vi "sav_dat2db.vi"(4 "Slide Ref":refnum<vi>, 6 "error in":errorcluster, 8 "Array":cluster{"x0":dbl, "dx":dbl, "y":sgl[][]}[](array[cluster]), 9 "date/time":timestamp) -> (1 "error out":errorcluster)   [LabVIEW 2010]
uses:
  <vilib>/addons/database/Auxilliary.llb/DB Tools Column Info.ctl
  <vilib>/addons/database/Auxilliary.llb/DB Tools DataTypes.ctl
  70user.lib/TheSigTab.vi
  <vilib>/addons/database/NI_Database_API.lvlib
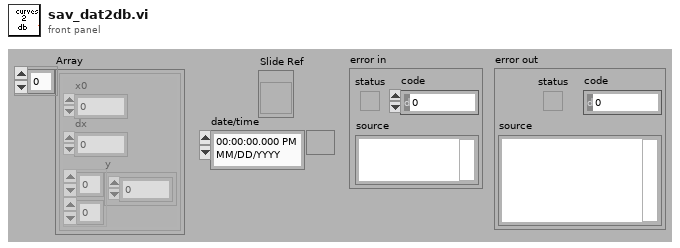
[diagram p1: front panel]
types:
  T1 = cluster{"type":string, "units":string, "n":i32}[]
  T2 = enum16{"Напряжение/Ток", "ЧР", "Температура", "Давление"}
  T3 = typedef "NI_Database_API.lvlib/DB Tools Column Info.ctl" = cluster{"column name":string, "data type":T4, "size":i32, "allow null?":bool}
  T4 = typedef "NI_Database_API.lvlib/DB Tools DataTypes.ctl" = enum16{"String", "Long (I32)", "Single (SGL)", "Double (DBL)", "Date/Time", "Binary"}
  T5 = typedef "NI_Database_API.lvlib/Conn ObjectReference.ctl" = refnum<k1>
  T6 = cluster{"Сигнал":string, "Тип":enum16{"Напряжение/Ток", "ЧР", "Температура", "Давление"}, "Object":string}[]
  T7 = cluster{"Сигнал":string, "Тип":enum16{"Напряжение/Ток", "ЧР", "Температура", "Давление"}, "Object":string}
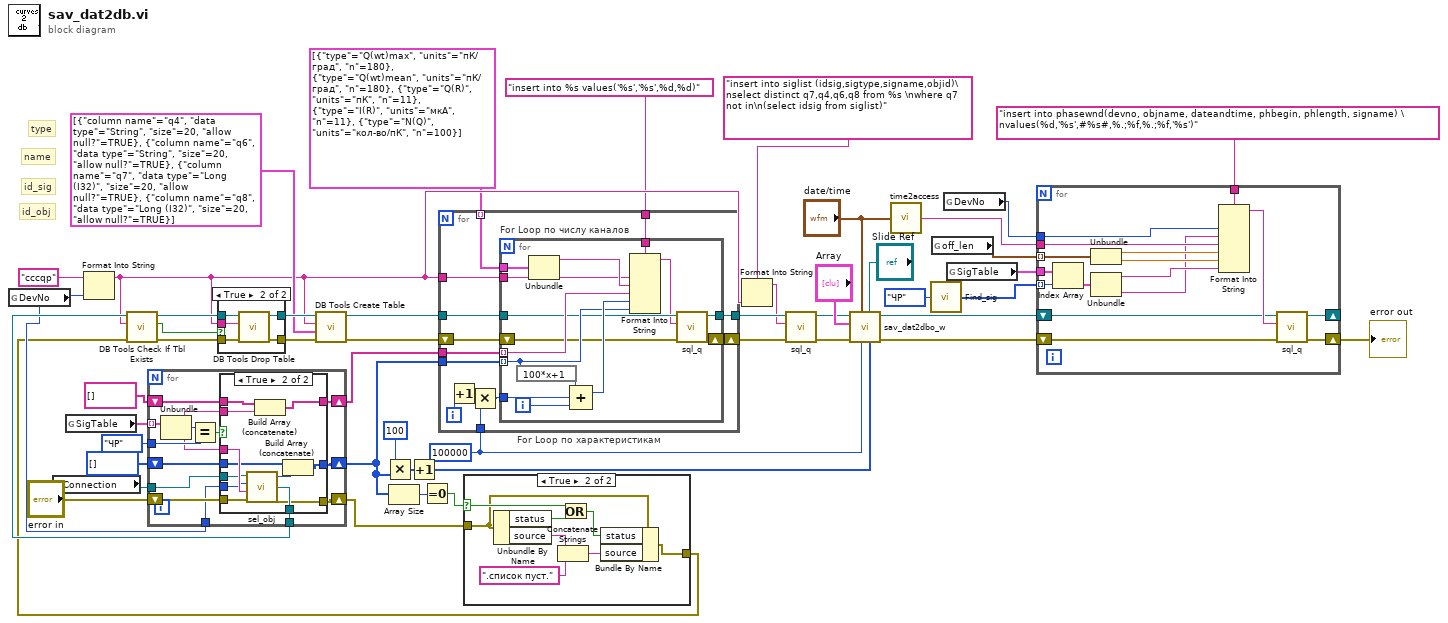
[diagram p0: block diagram]
diagram:
  w23 = 100000
  # "id_obj"
  # "id_sig"
  # "type"
  # "name"
  n1 = global read "TheSigTab.vi" "DevNo"() -> (w10:u32)
  n2 = global read "TheSigTab.vi" "Connection"() -> (w28:T5)
  n3 = global read "TheSigTab.vi" "SigTable"() -> (w48:T6)
  n4 = Format Into String(initial string="cccqp", w10) -> (resulting string=w31:string)  [unwired: 2 in, 1 out]
  n5 = for {
    tunnel: w48 -> [w59] mode=indexing
    shift-right: [w63] -> w46
    shift-left: string[] [] ("columns") -> [w62]
    tunnel: T2."ЧР" ("Тип") -> [w60]
    shift-right: [w56] -> w17
    shift-left: i32[] [] -> [w55]
    tunnel: w28 -> [w54]
    tunnel: [w53] -> w36
    shift-right: [w52] -> w1
    shift-left: "error in" -> [w51]
    tunnel: w10 -> [w50]
    n6 = Unbundle(w59) -> ("Сигнал"=w58:string, "Тип"=w64:T2, "Object"=w57:string)
    n7 = Equal?(x=w64, y=w60) -> (x = y?=w61:bool)
    n8 = case shown="True" w61 {
      tunnel: [w68 w80] -> w63
      tunnel: w62 -> [w68 w79]
      tunnel: w58 -> [_ w78]
      tunnel: w57 -> [_ w77]
      tunnel: [w67 w75] -> w56
      tunnel: w55 -> [w67 w74]
      tunnel: w54 -> [w66 w73]
      tunnel: [w66 w72] -> w53
      tunnel: [w65 w71] -> w52
      tunnel: w51 -> [w65 w70]
      tunnel: w50 -> [_ w69]
      frame False {
      }
      frame True {
        n9 = call "sel_obj.vi"("error in"=w70, "Object"=w77, "DevNo"=w69, "conn ref in"=w73) -> ("error out"=w71:errorcluster, "conn ref out"=w72:T5, "Obj Id"=w76:i32)
        n10 = Build Array (concatenate)(w79, w78) -> (w80:string[])
        n11 = Build Array (concatenate)(w74, w76) -> (w75:i32[])
      }
    }
  }
  n12 = Multiply(x=100, y=w17) -> (x*y=w44:i32[])
  n13 = Array Size(array=w17) -> (size(s)=w16:i32)
  n14 = Increment(x=w44) -> (x+1=w22:i32[])
  n15 = Equal To 0?(x=w16) -> (x = 0?=w2:bool)
  n16 = case shown="True" w2 {
    selector: w2 -> [_ w88]
    tunnel: [w81 w89] -> w3
    tunnel: w1 -> [w81 w86]
    frame False {
    }
    frame True {
      n17 = Unbundle By Name(w86) -> ("status"=w87:bool, "source"=w83:string)
      n18 = Concatenate Strings(w83, ".список пуст." ("source")) -> (w84:string)
      n19 = Or(x=w88, y=w87) -> (x .or. y?=w85:bool)
      n20 = Bundle By Name(cluster=w86, "status"=w85, "source"=w84) -> (w89:errorcluster)
    }
  }
  n21 = call <vilib>:"DB Tools Check If Tbl Exists.vi"("error in (no error)"=w3, "table name"=w31, "connection reference"=w36) -> ("error out"=w33:errorcluster, "exists?"=w34:bool, "connection reference out"=w35:T5)  [unwired: 2 in]
  n22 = case shown="True" w34 {
    tunnel: [w91 w96] -> w43
    tunnel: w31 -> [_ w95]
    tunnel: w35 -> [w91 w94]
    tunnel: w33 -> [w90 w93]
    tunnel: [w90 w92] -> w42
    frame False {
    }
    frame True {
      n23 = call <vilib>:"DB Tools Drop Table.vi"("error in (no error)"=w93, "table"=w95, "connection reference"=w94) -> ("error out"=w92:errorcluster, "connection reference out"=w96:T5)  [unwired: 5 in]
    }
  }
  n24 = call <vilib>:"DB Tools Create Table.vi"("error in (no error)"=w42, "column information"=T3[] [{"column name"="q4", "data type"=enum."String", "size"=20, "allow null?"=TRUE}, {"column name"="q6", "data type"=enum."String", "size"=20, "allow null?"=TRUE}, {"column name"="q7", "data type"=enum."Long (I32)", "size"=20, "allow null?"=TRUE}, {"column name"="q8", "data type"=enum."Long (I32)", "size"=20, "allow null?"=TRUE}], "table"=w31, "connection reference"=w43) -> ("error out"=w41:errorcluster, "connection reference out"=w40:T5)  [unwired: 4 in]
  n25 = for "For Loop по характеристикам" {
    shift-right: [w109] -> w20
    shift-left: w41 -> [w108]
    tunnel: w46 -> [w107]
    tunnel: w23 -> [w105]
    tunnel: w40 -> [w103]
    tunnel: w31 -> [w102]
    tunnel: [w101] -> w21
    tunnel: w17 -> [w100]
    tunnel: T1 [{"type"="Q(wt)max", "units"="пК/град", "n"=180}, {"type"="Q(wt)mean", "units"="пК/град", "n"=180}, {"type"="Q(R)", "units"="пК", "n"=11}, {"type"="I(R)", "units"="мкА", "n"=11}, {"type"="N(Q)", "units"="кол-во/пК", "n"=100}] -> [w98] mode=indexing
    tunnel: "insert into %s values('%s','%s',%d,%d)" -> [w97]
    i -> [w106]
    n26 = Increment(x=w106) -> (x+1=w104:i32)
    n27 = Multiply(x=w104, y=w105) -> (x*y=w99:i32)
    n28 = for "For Loop по числу каналов" {
      shift-right: [w113] -> w109
      shift-left: w108 -> [w112]
      tunnel: w107 -> [w120] mode=indexing
      tunnel: w103 -> [w115]
      tunnel: w102 -> [w116]
      tunnel: [w114] -> w101
      tunnel: w100 -> [w118] mode=indexing
      tunnel: w99 -> [w124]
      tunnel: w98 -> [w121]
      tunnel: w97 -> [w110]
      i -> [w123]
      n29 = expression code="100*x+1"(w118) -> (w122:i32)
      n30 = Unbundle(w121) -> ("type"=w117:string)  [unwired: 2 out]
      n31 = Compound Arithmetic op=ADD(w122, w124, w123) -> (w119:i32)
      n32 = Format Into String(format string=w110, w116, w117, w120, w119, w118) -> (resulting string=w111:string)  [unwired: 2 in, 1 out]
      n33 = call "sql_q.vi"("error in"=w112, "SQL query"=w111, "connect ref"=w115) -> ("error out"=w113:errorcluster, "conn ref out"=w114:T5)  [unwired: 1 in, 2 out]
    }
  }
  n34 = Format Into String(format string="insert into siglist (idsig,sigtype,signame,objid)\nselect distinct q7,q4,q6,q8 from %s \nwhere q7 not in\n(select idsig from siglist)", w31) -> (resulting string=w9:string)  [unwired: 2 in, 1 out]
  n35 = call "sql_q.vi"("error in"=w20, "SQL query"=w9, "connect ref"=w21) -> ("error out"=w18:errorcluster, "conn ref out"=w19:T5)  [unwired: 1 in, 2 out]
  n36 = call "sav_dat2dbo_w.vi"("ObjIds"=w22, "Slide Ref"="Slide Ref", "Mult"=w23, "date/time"="date/time", "error in"=w18, "Array"="Array", "conn ref"=w19) -> ("error out"=w24:errorcluster, "conn ref out"=w25:T5)  [unwired: 3 in]
  n37 = call "time2access.vi"("time stamp"="date/time") -> ("date/time string"=w4:string)
  n38 = call "Find_sig.vi"("Тип"=T2."ЧР") -> ("Indexies"=w11:i32[])
  n39 = global read "TheSigTab.vi" "off_len"() -> (w13:cluster{"offset":dbl, "length":dbl}[])
  n40 = global read "TheSigTab.vi" "DevNo"() -> (w14:u32)
  n41 = global read "TheSigTab.vi" "SigTable"() -> (w12:T6)
  n42 = for {
    shift-right: [w131] -> w29
    shift-left: w24 -> [w126]
    shift-right: [w130] -> _
    shift-left: w25 -> [w127]
    tunnel: w14 -> [w128]
    tunnel: w13 -> [w140] mode=indexing
    tunnel: w12 -> [w139]
    tunnel: w11 -> [w137] mode=indexing
    tunnel: w4 -> [w135]
    tunnel: "insert into phasewnd(devno, objname, dateandtime, phbegin, phlength, signame) \nvalues(%d,'%s',#%s#,%.;%f,%.;%f,'%s')" -> [w136]
    n43 = Index Array(array=w139, index=w137) -> (element=w138:T7)
    n44 = Unbundle(w140) -> ("offset"=w134:dbl, "length"=w133:dbl)
    n45 = Unbundle(w138) -> ("Сигнал"=w132:string, "Object"=w125:string)  [unwired: 1 out]
    n46 = Format Into String(format string=w136, w128, w125, w135, w134, w133, w132) -> (resulting string=w129:string)  [unwired: 2 in, 1 out]
    n47 = call "sql_q.vi"("error in"=w126, "SQL query"=w129, "connect ref"=w127) -> ("error out"=w131:errorcluster, "conn ref out"=w130:T5)  [unwired: 1 in, 2 out]
  }
  "error out" <- w29
